vi "Laco_iteracao.vi"() -> ()   [LabVIEW 2020]
panel:
  in  "stop":bool
  out "Numeric":dbl
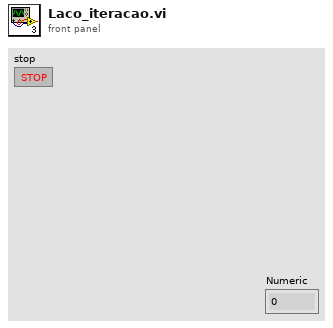
[diagram p1: front panel]
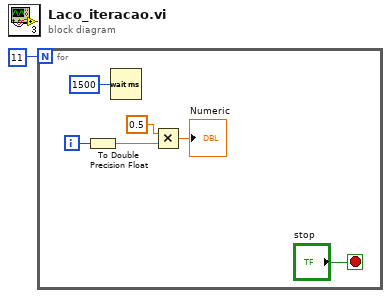
[diagram p0: block diagram]
diagram:
  n1 = for {
    N: 11 -> [_]
    i -> [w4]
    stop <- "stop" stop-if-true
    n2 = To Double Precision Float(number=w4) -> (double precision float=w3:dbl)
    n3 = Wait (ms)(milliseconds to wait=u32 1500) -> ()  [unwired: 1 out]
    n4 = Multiply(x=0.5, y=w3) -> (x*y=→"Numeric":dbl)
  }
